vi "Configure Output Regulation.vi"(0 "VISA resource name":refnum<visa-resource-name>, 5 "Channel Name (1)":string="1", 9 "Output Regulation Priority (1: Voltage)":i32(ring)=1 items=["Voltage"=1, "Current"=0], 11 "error in (no error)":errorcluster {"code" format="%.0x"}) -> (4 "VISA resource name out":refnum<visa-resource-name>, 15 "error out":errorcluster {"code" format="%.0x"})   [LabVIEW 2010, in "Agilent N6700 Series.lvlib"]
doc: "Selects whether the output regulation is in voltage or current priority mode.\n\n<b>Note:</b>\n\nThis VI only applies to models N678xA SMU."
uses:
  Agilent N6700 Series.lvlib
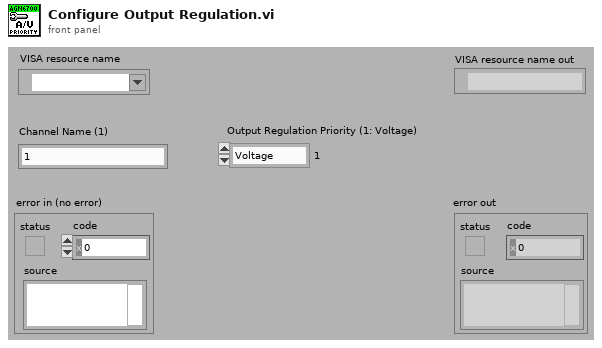
[diagram p1: front panel]
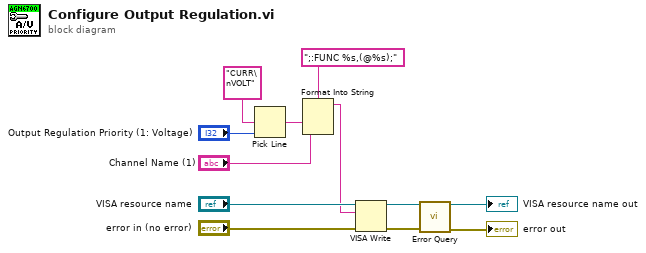
[diagram p0: block diagram]
diagram:
  n1 = Pick Line(multi-line string="CURR\nVOLT", line index="Output Regulation Priority (1: Voltage)") -> (output string=w3:string)  [unwired: 1 in]
  n2 = Format Into String(format string=";:FUNC %s,(@%s);", w3, "Channel Name (1)") -> (resulting string=w2:string)  [unwired: 2 in, 1 out]
  n3 = VISA Write(VISA resource name="VISA resource name", write buffer=w2, error in (no error)="error in (no error)") -> (VISA resource name out=w8:refnum<visa-resource-name>, error out=w7:errorcluster)  [unwired: 1 out]
  n4 = call "Error Query.vi"("VISA resource name"=w8, "error in (no error)"=w7) -> ("VISA resource name out"=→"VISA resource name out":refnum<visa-resource-name>, "error out"=→"error out":errorcluster)  [unwired: 10 in, 2 out]
